vi "niScope Abort.vi"(0 "instrument handle":refnum<k15>, 11 "error in":errorcluster) -> (4 "instrument handle out":refnum<k15>, 15 "error out":errorcluster)   [LabVIEW 2013]
doc: "Aborts an acquisition without changing the settings on the digitizer. Use this VI if the digitizer times out waiting for a trigger."
uses:
  niScope_32.dll
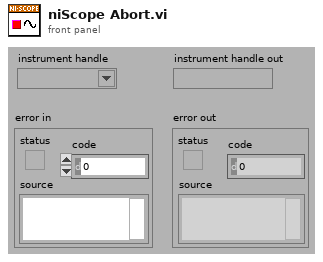
[diagram p1: front panel]
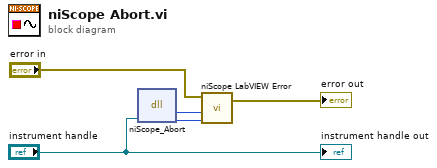
[diagram p0: block diagram]
diagram:
  n1 = dll-call lib="niScope_*.*" fn="niScope_Abort"("instrument handle"="instrument handle") -> ("status"=w2:i32, "instrument handle"=w3:u32)  [unwired: 3 in, 2 out]
  n2 = call <instrlib>:"niScope LabVIEW Error.vi"("instrument handle"=w3, "niScope error code (0)"=w2, "error in (no error)"="error in") -> ("error out"=→"error out":errorcluster)  [unwired: 2 in]
  "instrument handle out" <- "instrument handle"
